vi "TrajectoryState_Interpolate.vi"(6 "interpolantFraction":dbl, 9 "endValueTRAJ_STATE":T1={"TimeSeconds"=0.0, "Velocity"=0.0, "Acceleration"=0.0, "POSE"={"TRANSLATION"={"X"=0.0, "Y"=0.0}, "ROTATION"={"VALUE"=0.0, "COS"=1.0, "SIN"=0.0}}, "Curvature"=0.0} {"POSE"."ROTATION"."SIN" format="%13.4f"; "POSE"."ROTATION"."COS" format="%13.4f"; "POSE"."ROTATION"."VALUE" format="%13.4f"; "POSE"."TRANSLATION"."Y" format="%14.3f"; "POSE"."TRANSLATION"."X" format="%14.3f"}, 11 "inputTRAJ_STATE":T1={"TimeSeconds"=0.0, "Velocity"=0.0, "Acceleration"=0.0, "POSE"={"TRANSLATION"={"X"=0.0, "Y"=0.0}, "ROTATION"={"VALUE"=0.0, "COS"=1.0, "SIN"=0.0}}, "Curvature"=0.0} {"POSE"."ROTATION"."SIN" format="%13.4f"; "POSE"."ROTATION"."COS" format="%13.4f"; "POSE"."ROTATION"."VALUE" format="%13.4f"; "POSE"."TRANSLATION"."Y" format="%14.3f"; "POSE"."TRANSLATION"."X" format="%14.3f"}) -> (3 "OutputTRAJ_STATE":T1={"TimeSeconds"=0.0, "Velocity"=0.0, "Acceleration"=0.0, "POSE"={"TRANSLATION"={"X"=0.0, "Y"=0.0}, "ROTATION"={"VALUE"=0.0, "COS"=1.0, "SIN"=0.0}}, "Curvature"=0.0} {"POSE"."ROTATION"."SIN" format="%13.4f"; "POSE"."ROTATION"."COS" format="%13.4f"; "POSE"."ROTATION"."VALUE" format="%13.4f"; "POSE"."TRANSLATION"."Y" format="%14.3f"; "POSE"."TRANSLATION"."X" format="%14.3f"})   [LabVIEW 2019, in "Trajectory_Library.lvlib"]
doc: "Interpolates between two States.\n \nParameters:\n - inputTrajState - The current trajectory state data structure\n - endValueTrajState - The end value for the interpolation.\n - interpolantFactor - The interpolant (fraction).\n\nReturns:\n - TrajState - The interpolated state."
uses:
  Trajectory_Library.lvlib
  TypeDef/TRANSLATION2D.ctl
  TypeDef/ROTATION2D.ctl
  TypeDef/POSE2D.ctl
  TypeDef/TRAJ_STATE.ctl
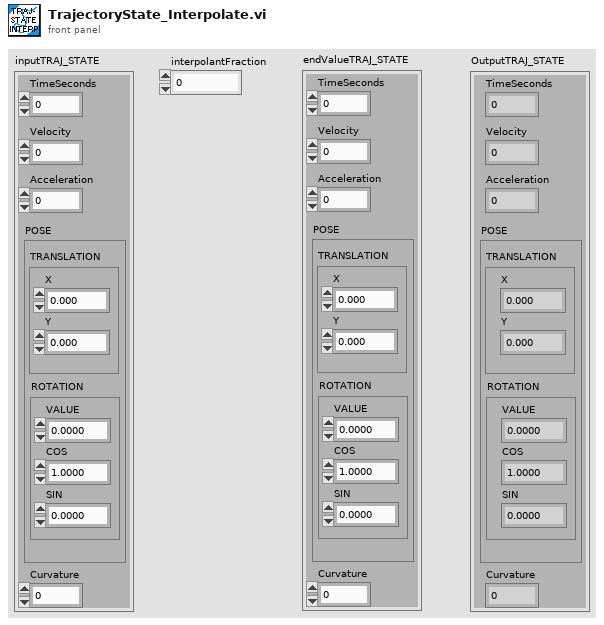
[diagram p1: front panel]
types:
  T1 = typedef "Trajectory_Library.lvlib/TRAJ_STATE.ctl" = cluster{"TimeSeconds":dbl, "Velocity":dbl, "Acceleration":dbl, "POSE":T2, "Curvature":dbl}
  T2 = typedef "Trajectory_Library.lvlib/POSE2D.ctl" = cluster{"TRANSLATION":T3, "ROTATION":T4}
  T3 = typedef "Trajectory_Library.lvlib/TRANSLATION2D.ctl" = cluster{"X":dbl, "Y":dbl}
  T4 = typedef "Trajectory_Library.lvlib/ROTATION2D.ctl" = cluster{"VALUE":dbl, "COS":dbl, "SIN":dbl}
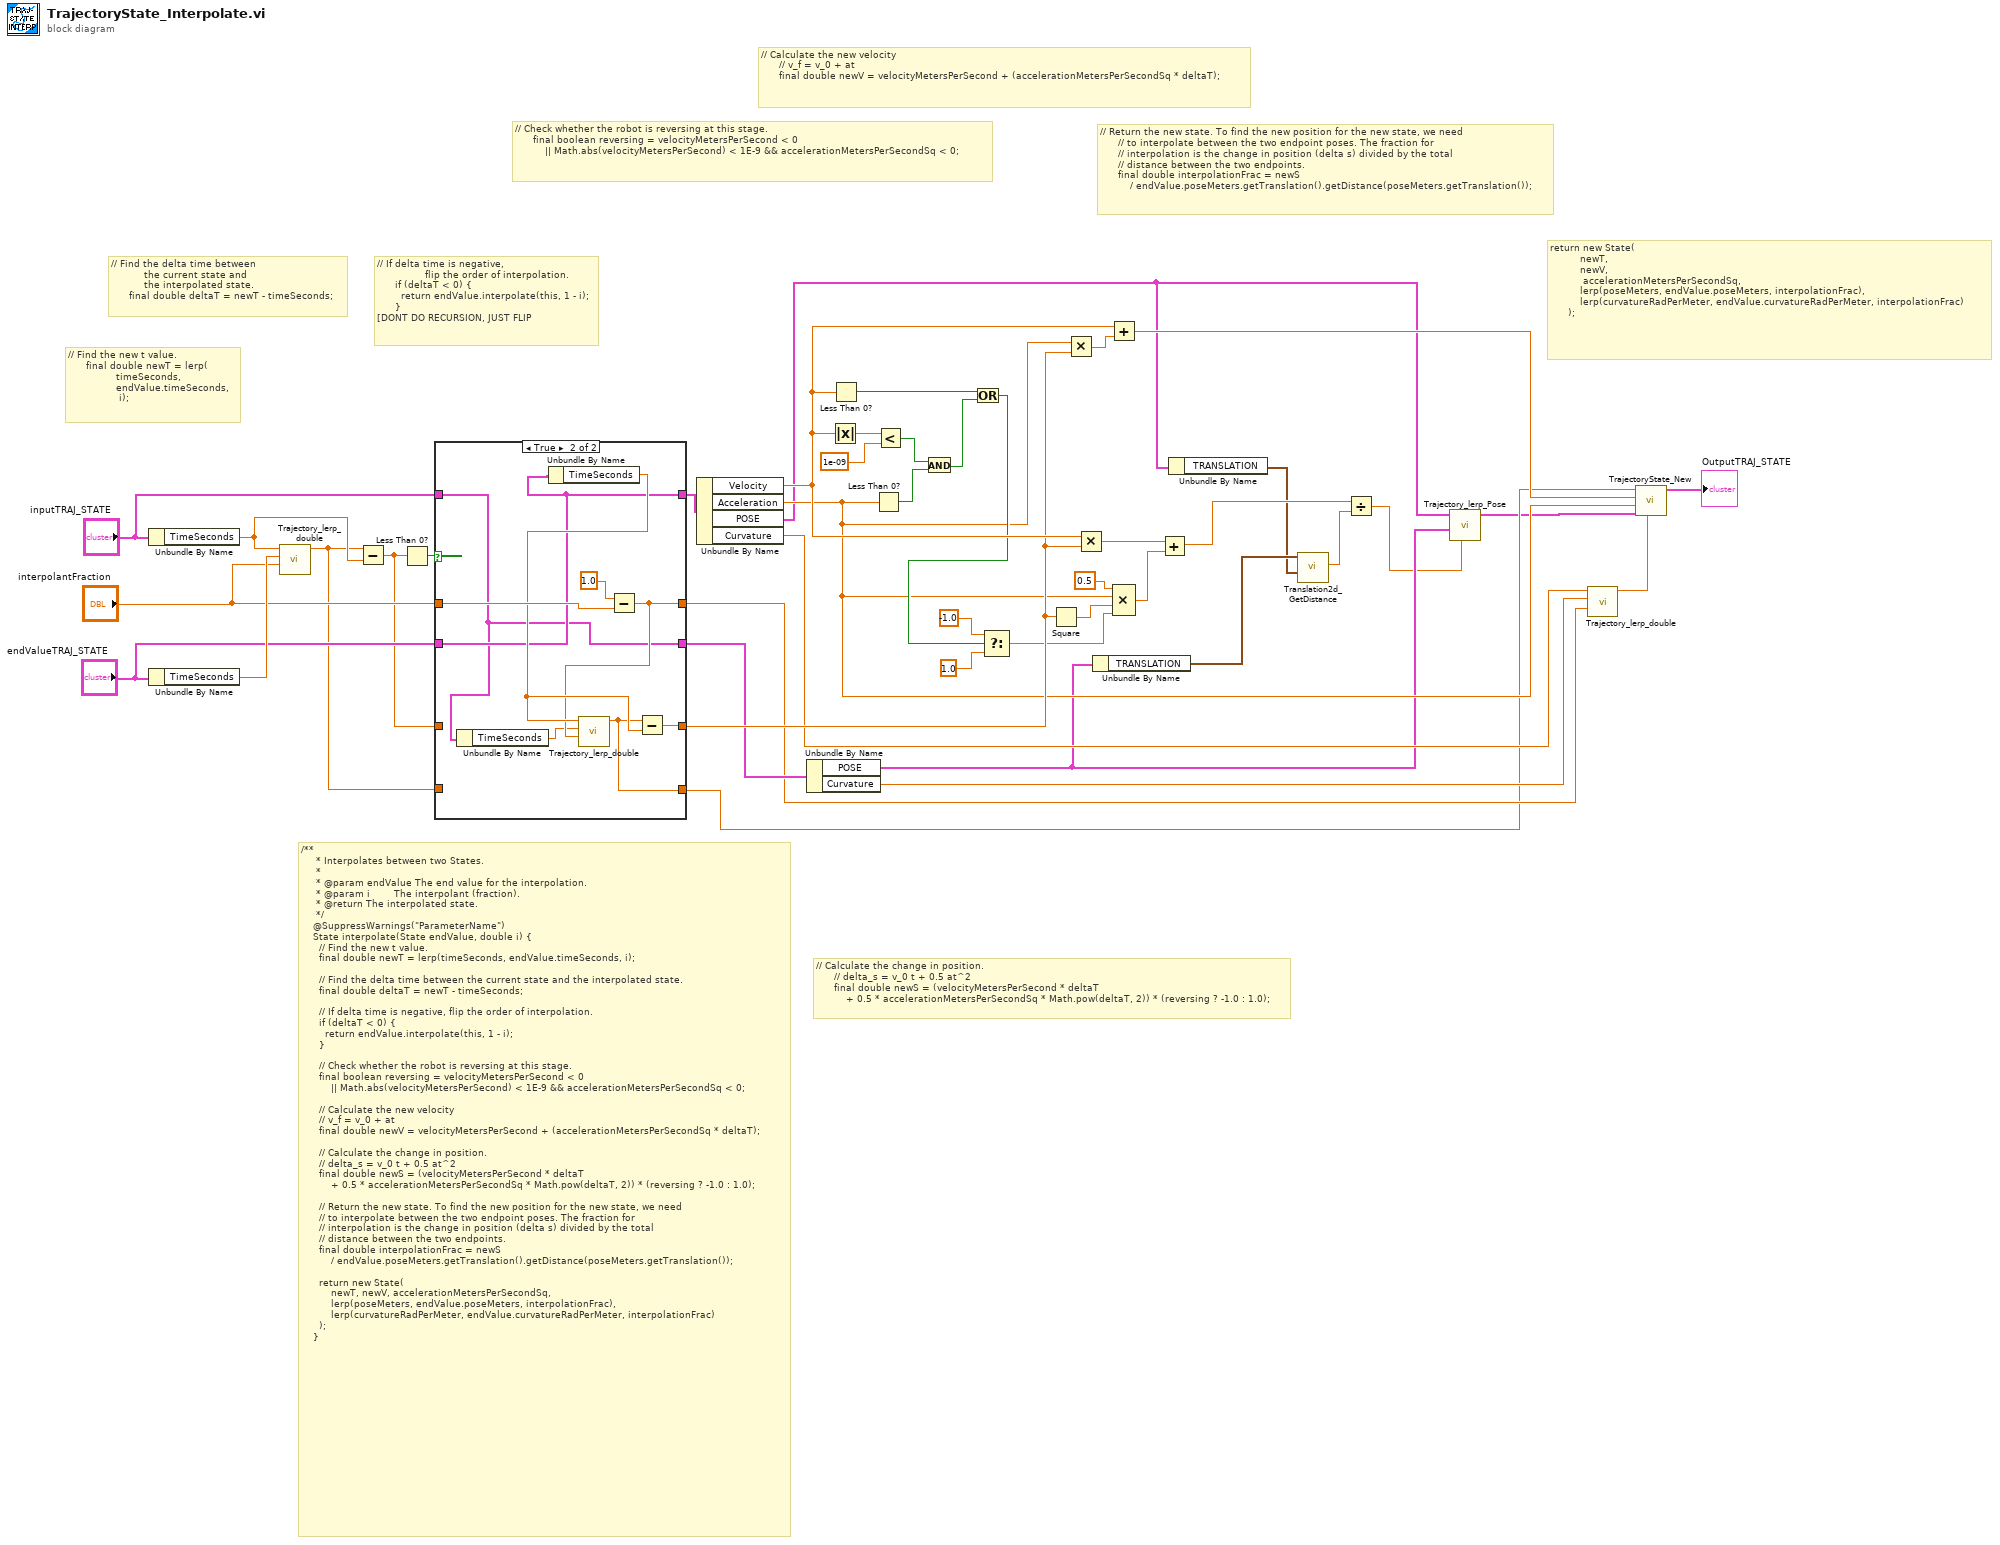
[diagram p0: block diagram]
diagram:
  # "return new State(\n          newT, \n          newV, \n           accelerationMetersPerSecondSq,\n          lerp(poseMeters, endValue.poseMeters, interpolationFrac),\n          lerp(curvatureRadPerMeter, endValue.curvatureRadPerMeter, interpolationFrac)\n      );"
  # "// Return the new state. To find the new position for the new state, we need\n      // to interpolate between the two endpoint poses. The fraction for\n      // interpolation is the change in position (delta s) divided by the total\n      // distance between the two endpoints.\n      final double interpolationFrac = newS\n          / endValue.poseMeters.getTranslation().getDistance(poseMeters.getTranslation());"
  # "// Calculate the change in position.\n      // delta_s = v_0 t + 0.5 at^2\n      final double newS = (velocityMetersPerSecond * deltaT\n          + 0.5 * accelerationMetersPerSecondSq * Math.pow(deltaT, 2)) * (reversing ? -1.0 : 1.0);"
  # "// Calculate the new velocity\n      // v_f = v_0 + at\n      final double newV = velocityMetersPerSecond + (accelerationMetersPerSecondSq * deltaT);"
  # "// Check whether the robot is reversing at this stage.\n      final boolean reversing = velocityMetersPerSecond < 0\n          || Math.abs(velocityMetersPerSecond) < 1E-9 && accelerationMetersPerSecondSq < 0;"
  # "// If delta time is negative, \n                flip the order of interpolation.\n      if (deltaT < 0) {\n        return endValue.interpolate(this, 1 - i);\n      }\n[DONT DO RECURSION, JUST FLIP"
  # "// Find the delta time between \n           the current state and \n           the interpolated state.\n      final double deltaT = newT - timeSeconds;"
  # "// Find the new t value.\n      final double newT = lerp(\n                timeSeconds, \n                endValue.timeSeconds, \n                 i);"
  # "/**\n     * Interpolates between two States.\n     *\n     * @param endValue The end value for the interpolation.\n     * @param i        The interpolant (fraction).\n     * @return The interpolated state.\n     */\n    @SuppressWarnings(\"ParameterName\")\n    State interpolate(State endValue, double i) {\n      // Find the new t value.\n      final double newT = lerp(timeSeconds, endValue.timeSeconds, i);\n\n      // Find the delta time between the current state and the interpolated state.\n      final double deltaT = newT - timeSeconds;\n\n      // If delta time is negative, flip the order of interpolation.\n      if (deltaT < 0) {\n        return endValue.interpolate(this, 1 - i);\n      }\n\n      // Check whether the robot is reversing at this stage.\n      final boolean reversing = velocityMetersPerSecond < 0\n          || Math.abs(velocityMetersPerSecond) < 1E-9 && accelerationMetersPerSecondSq < 0;\n\n      // Calculate the new velocity\n      // v_f = v_0 + at\n      final double newV = velocityMetersPerSecond + (accelerationMetersPerSecondSq * deltaT);\n\n      // Calculate the change in position.\n      // delta_s = v_0 t + 0.5 at^2\n      final double newS = (velocityMetersPerSecond * deltaT\n          + 0.5 * accelerationMetersPerSecondSq * Math.pow(deltaT, 2)) * (reversing ? -1.0 : 1.0);\n\n      // Return the new state. To find the new position for the new state, we need\n      // to interpolate between the two endpoint poses. The fraction for\n      // interpolation is the change in position (delta s) divided by the total\n      // distance between the two endpoints.\n      final double interpolationFrac = newS\n          / endValue.poseMeters.getTranslation().getDistance(poseMeters.getTranslation());\n\n      return new State(\n          newT, newV, accelerationMetersPerSecondSq,\n          lerp(poseMeters, endValue.poseMeters, interpolationFrac),\n          lerp(curvatureRadPerMeter, endValue.curvatureRadPerMeter, interpolationFrac)\n      );\n    }"
  n1 = Unbundle By Name("inputTRAJ_STATE") -> ("TimeSeconds"=w42:dbl)
  n2 = Unbundle By Name("endValueTRAJ_STATE") -> ("TimeSeconds"=w43:dbl)
  n3 = call "Trajectory_lerp_double.vi"("fraction"="interpolantFraction", "endValue"=w43, "startValue"=w42) -> ("outputValue"=w10:dbl)  [unwired: 8 in]
  n4 = Subtract(x=w10, y=w42) -> (x-y=w30:dbl)
  n5 = Less Than 0?(x=w30) -> (x < 0?=w41:bool)
  n6 = case shown="True" w41 {
    tunnel: [w48 w51] -> w37
    tunnel: "inputTRAJ_STATE" -> [w48 w50]
    tunnel: [w47 w50] -> w14
    tunnel: "endValueTRAJ_STATE" -> [w47 w51]
    tunnel: [w46 w53] -> w12
    tunnel: "interpolantFraction" -> [w46 w56]
    tunnel: w30 -> [w45 _]
    tunnel: [w45 w55] -> w25
    tunnel: w10 -> [w44 _]
    tunnel: [w44 w49] -> w9
    frame False {
    }
    frame True {
      n7 = Unbundle By Name(w50) -> ("TimeSeconds"=w52:dbl)
      n8 = Unbundle By Name(w51) -> ("TimeSeconds"=w54:dbl)
      n9 = Subtract(x=1.0, y=w56) -> (x-y=w53:dbl)
      n10 = call "Trajectory_lerp_double.vi"("fraction"=w53, "endValue"=w52, "startValue"=w54) -> ("outputValue"=w49:dbl)  [unwired: 8 in]
      n11 = Subtract(x=w49, y=w54) -> (x-y=w55:dbl)
    }
  }
  n12 = Unbundle By Name(w37) -> ("Velocity"=w28:dbl, "Acceleration"=w16:dbl, "POSE"=w3:T2, "Curvature"=w15:dbl)
  n13 = Unbundle By Name(w14) -> ("POSE"=w5:T2, "Curvature"=w13:dbl)
  n14 = Absolute Value(x=w28) -> (abs(x)=w35:dbl)
  n15 = Less Than 0?(x=w28) -> (x < 0?=w36:bool)
  n16 = Less Than 0?(x=w16) -> (x < 0?=w32:bool)
  n17 = Less?(x=w35, y=1e-09) -> (x < y?=w33:bool)
  n18 = And(x=w33, y=w32) -> (x .and. y?=w31:bool)
  n19 = Or(x=w36, y=w31) -> (x .or. y?=w19:bool)
  n20 = Select(t=-1.0, s=w19, f=1.0) -> (s? t:f=w20:dbl)
  n21 = Square(x=w25) -> (x^2=w26:dbl)
  n22 = Multiply(x=w16, y=w25) -> (x*y=w29:dbl)
  n23 = Multiply(x=w28, y=w25) -> (x*y=w22:dbl)
  n24 = Unbundle By Name(w5) -> ("TRANSLATION"=w4:T3)
  n25 = Add(x=w28, y=w29) -> (x+y=w17:dbl)
  n26 = Compound Arithmetic op=MULTIPLY(0.5 ("value"), w16, w26, w20) -> (w21:dbl)
  n27 = Add(x=w22, y=w21) -> (x+y=w7:dbl)
  n28 = Unbundle By Name(w3) -> ("TRANSLATION"=w2:T3)
  n29 = call "Translation2d_GetDistance.vi"("other Translation"=w2, "In Translation"=w4) -> ("Distance"=w6:dbl)  [unwired: 9 in]
  n30 = Divide(x=w7, y=w6) -> (x/y=w1:dbl)
  n31 = call "Trajectory_lerp_Pose.vi"("interpolantFraction"=w1, "endPOSE"=w5, "startPOSE"=w3) -> ("outputPOSE"=w8:T2)  [unwired: 8 in]
  n32 = call "Trajectory_lerp_double.vi"("fraction"=w12, "endValue"=w13, "startValue"=w15) -> ("outputValue"=w11:dbl)  [unwired: 8 in]
  n33 = call "TrajectoryState_New.vi"("Curvature"=w11, "POSE"=w8, "Accel"=w16, "Velocity"=w17, "Time"=w9) -> ("TRAJ_STATE"=→"OutputTRAJ_STATE":T1)  [unwired: 6 in]
